vi "SetStringInfo.vi"(0 "reference":refnum<class "StateNode.lvclass">, 1 "State":string, 2 "Action":string, 5 "error in (no error)":errorcluster) -> (14 "reference out":refnum<class "StateNode.lvclass">, 19 "error out":errorcluster)   [LabVIEW 2016, in "StateNode.lvclass"]
uses:
  <resource>/Framework/Providers/Open_GDS/UML/StateNode_class/StateNode.lvclass
  <resource>/Framework/Providers/Open_GDS/UML/MultiLineString_class/MultiLineString.lvclass
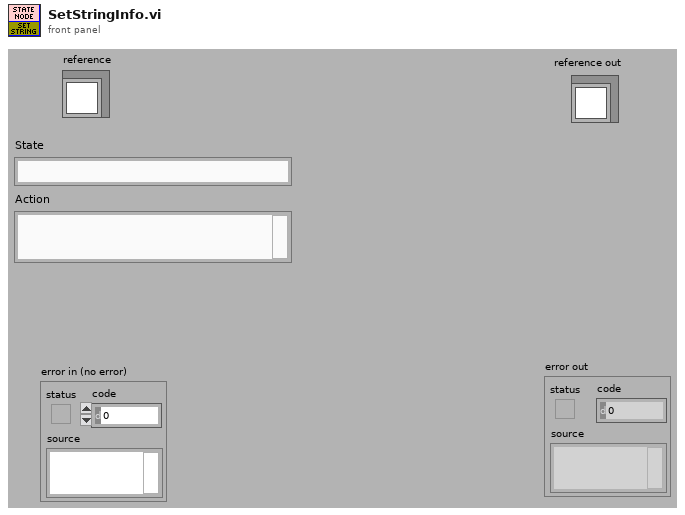
[diagram p1: front panel]
types:
  T1 = typedef "StateNode.lvclass/ObjectAttributes.ctl" = cluster{"state":refnum<class "MultiLineString.lvclass">, "action":refnum<class "MultiLineString.lvclass">, "DEFAULT_WIDTH":i32, "DEFAULT_HEIGHT":i32}
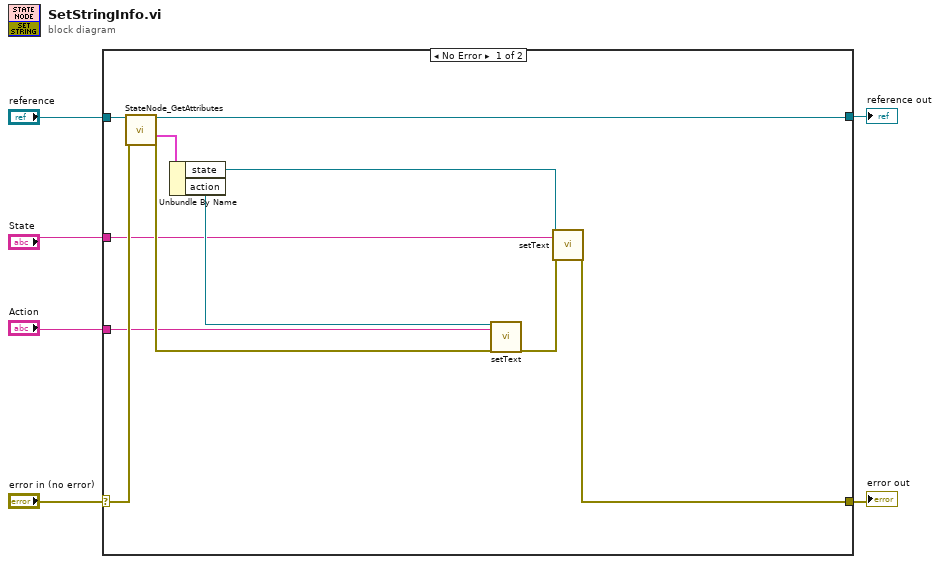
[diagram p0: block diagram]
diagram:
  n1 = case shown="No Error" "error in (no error)" {
    selector: "error in (no error)" -> [w17 w18]
    tunnel: "reference" -> [w16 w19]
    tunnel: [w10 w18] -> w4
    tunnel: [w15 w19] -> w3
    tunnel: "State" -> [w9 _]
    tunnel: "Action" -> [w8 _]
    frame No Error {
      n2 = call <resource>:"StateNode_GetAttributes.vi"("reference in"=w16, "error in (no error)"=w17) -> ("reference out"=w15:refnum<class "StateNode.lvclass">, "Data"=w7:T1, "error out"=w11:errorcluster)  [unwired: 1 in, 14 out]
      n3 = Unbundle By Name(w7) -> ("state"=w13:refnum<class "MultiLineString.lvclass">, "action"=w12:refnum<class "MultiLineString.lvclass">)
      n4 = call-dynamic "setText.vi"("reference"=w12, "text"=w8, "error in (no error)"=w11) -> ("error out"=w14:errorcluster)  [unwired: 16 out]
      n5 = call-dynamic "setText.vi"("reference"=w13, "text"=w9, "error in (no error)"=w14) -> ("error out"=w10:errorcluster)  [unwired: 16 out]
    }
    frame Error {
    }
  }
  "reference out" <- w3
  "error out" <- w4
